vi "gentec-SOLO-PE.set Correction.vi"(8 "error in (no error)":errorcluster, 9 "Correction Value":dbl, 10 "Correction Type":T1 items=["Multiplier1", "Offset 1", "Multiplier 2", "Offset 2"], 11 "VISA Refnum in":refnum<visa-resource-name>) -> (0 "error out":errorcluster, 1 "Acknoledged?":bool, 2 "Error":string, 3 "VISA Refnum out":refnum<visa-resource-name>, 4 "Timeout":bool)   [LabVIEW 2014, in "gentec-SOLO-PE - Driver.lvlib"]
doc: "Sets correction values for Offset and Multipliers."
uses:
  gentec-SOLO-PE - Driver.lvlib
  Type Defs/gentec-SOLO-PE.Correction Type.ctl
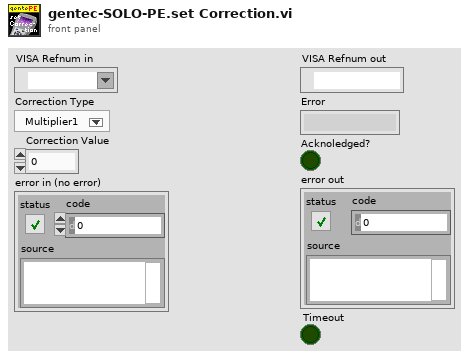
[diagram p1: front panel]
types:
  T1 = typedef "gentec-SOLO-PE - Driver.lvlib/gentec-SOLO-PE.Correction Type.ctl" = u16
  T2 = typedef "gentec-SOLO-PE - Driver.lvlib/gentec-SOLO-PE.Scale.ctl" = u32
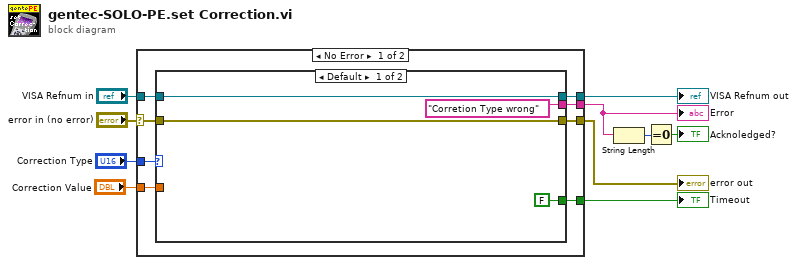
[diagram p0: block diagram]
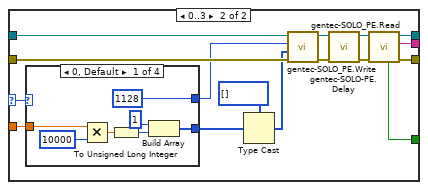
[diagram p2: hidden frame]
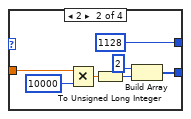
[diagram p3: hidden frame]
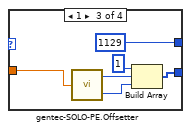
[diagram p4: hidden frame]
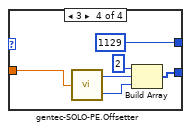
[diagram p5: hidden frame]
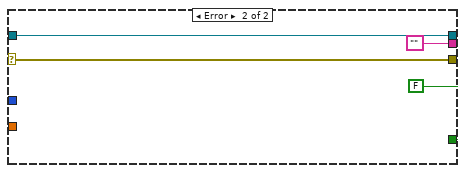
[diagram p6: hidden frame]
diagram:
  n1 = case shown="No Error" "error in (no error)" {
    selector: "error in (no error)" -> [w15 w67]
    tunnel: [w13 w67] -> w10
    tunnel: [w18 w68] -> w9
    tunnel: [w14 ""] -> w4
    tunnel: [w17 FALSE ("Timeout")] -> w8
    tunnel: "VISA Refnum in" -> [w16 w68]
    tunnel: "Correction Type" -> [w11 _]
    tunnel: "Correction Value" -> [w12 _]
    frame No Error {
      n2 = case shown="Default" w11 {
        selector: w11 -> [_ w23]
        tunnel: [w22 w38] -> w18
        tunnel: [FALSE ("Timeout") w37] -> w17
        tunnel: w16 -> [w22 w32]
        tunnel: w15 -> [w21 w31]
        tunnel: ["Corretion Type wrong" ("Error") w30] -> w14
        tunnel: [w21 w29] -> w13
        tunnel: w12 -> [_ w26]
        frame Default {
        }
        frame 0..3 {
          n3 = case shown="0, Default" w23 {
            tunnel: w26 -> [w44 w51 w55 w61]
            tunnel: [w41 w48 w57 w63] -> w25
            tunnel: [u16 1128 ("Command Handle") u16 1128 ("Command Handle") u16 1129 ("Command Handle") u16 1129 ("Command Handle")] -> w24
            frame 0, Default {
              n4 = Multiply(x=w44, y=10000) -> (x*y=w42:dbl)
              n5 = To Unsigned Long Integer(number=w42) -> (unsigned 32bit integer=w39:u32)
              n6 = Build Array(u32 1, w39) -> (w41:u32[])
            }
            frame 2 {
              n7 = Multiply(x=w51, y=10000) -> (x*y=w49:dbl)
              n8 = To Unsigned Long Integer(number=w49) -> (unsigned 32bit integer=w46:u32)
              n9 = Build Array(u32 2, w46) -> (w48:u32[])
            }
            frame 1 {
              n10 = call "gentec-SOLO-PE.Offsetter.vi"("Value"=w55) -> ("Value"=w54:u32, "Scale"=w53:T2)
              n11 = Build Array(u32 1, w54, w53) -> (w57:T2[])
            }
            frame 3 {
              n12 = call "gentec-SOLO-PE.Offsetter.vi"("Value"=w61) -> ("Value"=w60:u32, "Scale"=w59:T2)
              n13 = Build Array(u32 2, w60, w59) -> (w63:T2[])
            }
          }
          n14 = Type Cast(type=u32[] [], x=w25) -> (*(type *) &x=w27:u32[])
          n15 = call "gentec-SOLO_PE.Write.vi"("error in (no error)"=w31, "Parameters (Empty)"=w27, "Command Handle"=w24, "VISA Refnum in"=w32) -> ("error out"=w35:errorcluster, "VISA Refnum out"=w33:refnum<visa-resource-name>)  [unwired: 6 in]
          n16 = call "gentec-SOLO-PE.Delay.vi"("error in (no error)"=w35, "VISA resource In"=w33) -> ("error out"=w36:errorcluster, "VISA resource Out"=w34:refnum<visa-resource-name>)  [unwired: 4 in]
          n17 = call "gentec-SOLO_PE.Read.vi"("error in (no error)"=w36, "VISA Refnum in"=w34) -> ("error out"=w29:errorcluster, "Error"=w30:string, "VISA Refnum out"=w38:refnum<visa-resource-name>, "Timeout"=w37:bool)  [unwired: 5 in, 1 out]
        }
      }
    }
    frame Error {
    }
  }
  "error out" <- w10
  "VISA Refnum out" <- w9
  "Error" <- w4
  "Timeout" <- w8
  n18 = String Length(string=w4) -> (length=w3:i32)
  n19 = Equal To 0?(x=w3) -> (x = 0?=→"Acknoledged?":bool)
